vi "FilterCycle.vi"(7 "LabVIEW Web Service Request":refnum<class "Web Request.lvclass">, 9 "Length":u16, 10 "Period":u16, 11 "auto":u8) -> ()   [LabVIEW 2014]
uses:
  <vilib>/wsapi/Web Request.lvclass
  Controller/Messages/Update Filter State Params/Update Filter Cycle Params MSG.lvclass
  Controller/Messages/Update Filter State Params/Update Filter Cycle Params MSG.lvclass/Update Filter Cycle Params MSG.ctl
  Controller/Messages/Update Filter State Params/Write Cycle_.vi
  Controller/Messages/Update Filter State Params/Write Length.vi
  Controller/Messages/Update Filter State Params/Write Period.vi
  Controller/Controller.lvclass
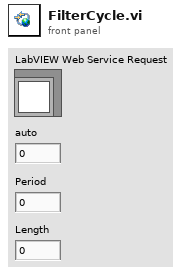
[diagram p1: front panel]
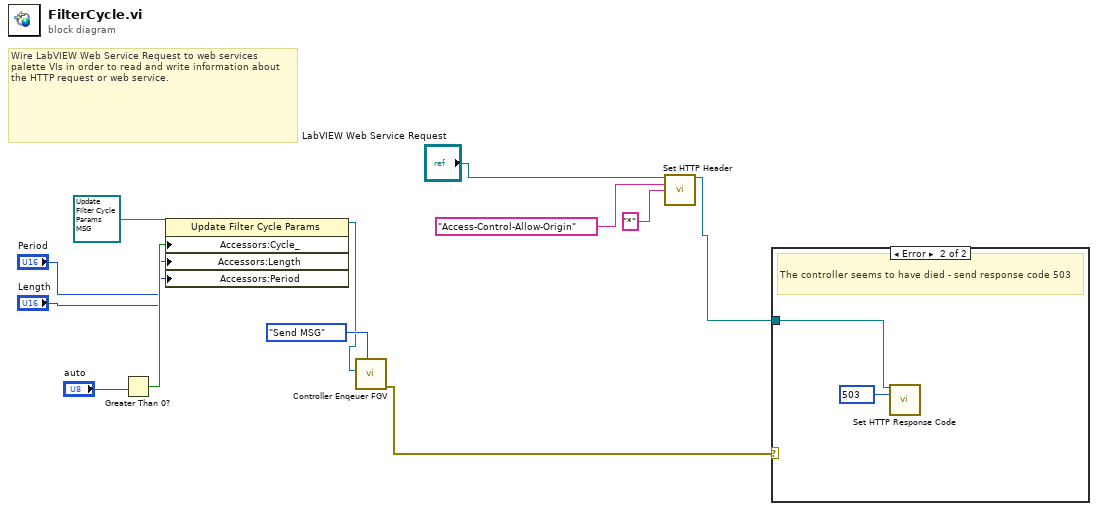
[diagram p0: block diagram]
diagram:
  # "Wire LabVIEW Web Service Request to web services palette VIs in order to read and write information about the HTTP request or web service."
  n1 = Greater Than 0?(x="auto") -> (x > 0?=w9:bool)
  n2 = property class="Update Filter Cycle Params"(reference=refnum<class "Update Filter Cycle Params MSG.lvclass"> refnum ("Controller.lvlib:Update Filter Cycle Params"), "Accessors:Cycle_"=w9, "Accessors:Length"="Length", "Accessors:Period"="Period") -> (reference out=w6:refnum<class "Update Filter Cycle Params MSG.lvclass">)  [unwired: 1 in, 1 out]
  n3 = call "Controller Enqeuer FGV.vi"("State"=enum16{"Store", "Send MSG"}."Send MSG", "MSG"=w6) -> ("error out"=w2:errorcluster)  [unwired: 9 in]
  n4 = call <vilib>:"Set HTTP Header.vi"("LabVIEW Web Service Request"="LabVIEW Web Service Request", "header"="Access-Control-Allow-Origin", "header value"="*") -> ("LabVIEW Web Service Request out"=w1:refnum<class "Web Request.lvclass">)  [unwired: 11 in, 1 out]
  n5 = case shown="Error" w2 {
    tunnel: w1 -> [_ w13]
    frame No Error {
    }
    frame Error {
      w14 = 503 items=["100"=100, "101"=101, "200"=200, "201"=201, "202"=202, "203"=203, "204"=204, "205"=205, "206"=206, "300"=300, "301"=301, "302"=302, "303"=303, "304"=304, "305"=305, "306"=306, "307"=307, "400"=400, "401"=401, "402"=402, "403"=403, "404"=404, "405"=405, "406"=406, "407"=407, "408"=408, "409"=409, "410"=410, "411"=411, "412"=412, "413"=413, "414"=414, "415"=415, "416"=416, "417"=417, "500"=500, "501"=501, "502"=502, "503"=503, "504"=504, "505"=505] ("response code (200)")
      # "The controller seems to have died - send response code 503"
      n6 = call <vilib>:"Set HTTP Response Code.vi"("LabVIEW Web Service Request"=w13, "response code (200)"=w14) -> ()  [unwired: 12 in, 2 out]
    }
  }
